vi "TCam_FixpointTemps.vi"(2 "input cluster":T1={"Core"={"Current VI Reference"=refnum, "Close Panel on Exit?"=FALSE}, "Image Out"=refnum, "State"=0, "Points"={"Top Left"={"X"=0.0, "Y"=0.0}, "Top Right"={"X"=0.0, "Y"=0.0}, "Bottom Left"={"X"=0.0, "Y"=0.0}, "Bottom Right"={"X"=0.0, "Y"=0.0}, "x space 2"=0.0, "y space 2"=0.0, "x_space"=0.0, "y_space"=0.0, "Pixels"=[], "Fixpoint"={"X"=0.0, "Y"=0.0}}, "img_array"=[], "Temps"=[], "Temps_Array"=[], "Scan Area"=0.0, "Fixpoint Area"=0.0, "Config"={"Freezing"={"Cutoff"=2.0, "EndIndex"=2}}, "PCR Size"=0, "ImageCount"=0, "ShowGradient"=FALSE, "Save Well data"=FALSE, "Save Blackbody data"=FALSE, "Save Temps For Offset"=FALSE} {"Points"."Bottom Right"."Y" format="%.2f"; "Points"."Bottom Right"."X" format="%.2f"; "Points"."Top Left"."Y" format="%.2f"; "Points"."Top Left"."X" format="%.2f"; "Points"."Top Right"."Y" format="%.2f"; "Points"."Top Right"."X" format="%.2f"; "Points"."Bottom Left"."Y" format="%.2f"; "Points"."Bottom Left"."X" format="%.2f"; "Points"."Fixpoint"."Y" format="%.2f"; "Points"."Fixpoint"."X" format="%.2f"}, 3 "name or relative path":path, 4 "Therm_Temps":dbl[](array[numeric])) -> (0 "WellTemps":dbl[](array[numeric]), 1 "Offsets":dbl[](array[numeric]))   [LabVIEW 2024]
uses:
  DataCluster_TCAL.ctl
  <vilib>/vision/Image Controls.llb/IMAQ Image.ctl
  TCE_Config.ctl
  <vilib>/Utility/file.llb/Write Delimited Spreadsheet (DBL).vi
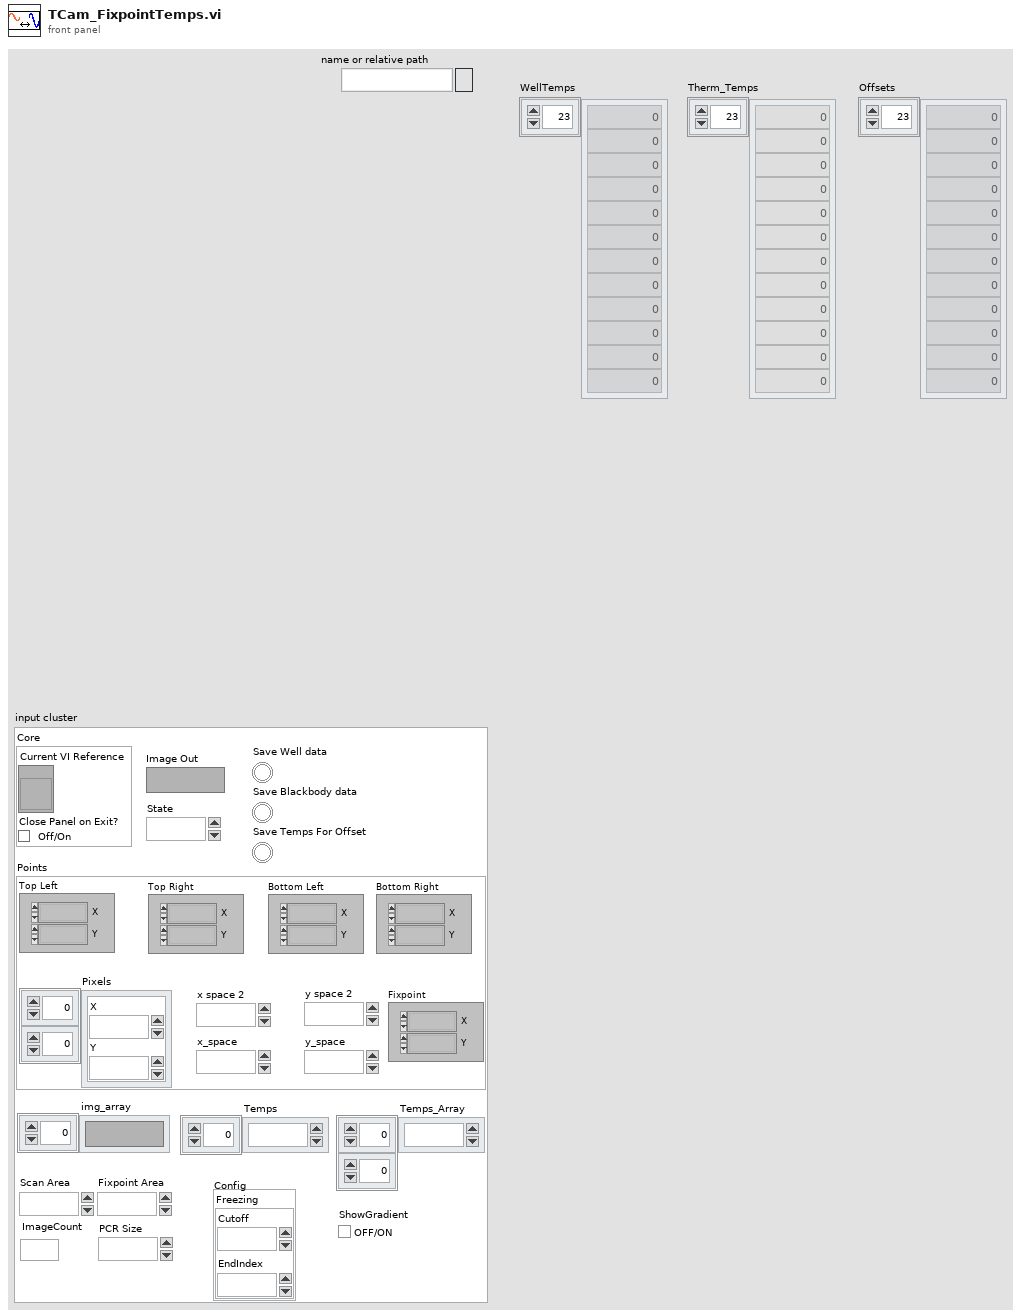
[diagram p1: front panel]
types:
  T1 = typedef "DataCluster_TCAL.ctl" = cluster{"Core":cluster{"Current VI Reference":refnum<vi>, "Close Panel on Exit?":bool}, "Image Out":T2, "State":i32, "Points":cluster{"Top Left":T3, "Top Right":T3, "Bottom Left":T3, "Bottom Right":T3, "x space 2":dbl, "y space 2":sgl, "x_space":sgl, "y_space":sgl, "Pixels":cluster{"X":i32, "Y":i32}[][], "Fixpoint":T3}, "img_array":T2[], "Temps":dbl[], "Temps_Array":dbl[][], "Scan Area":dbl, "Fixpoint Area":dbl, "Config":T4, "PCR Size":u16, "ImageCount":i32, "ShowGradient":bool, "Save Well data":bool, "Save Blackbody data":bool, "Save Temps For Offset":bool}
  T2 = typedef "IMAQ Image.ctl" = refnum<image>
  T3 = typedef "IMAQ Point" = cluster{"X":sgl, "Y":sgl}
  T4 = typedef "TCE_Config.ctl" = cluster{"Freezing":cluster{"Cutoff":dbl, "EndIndex":i32}}
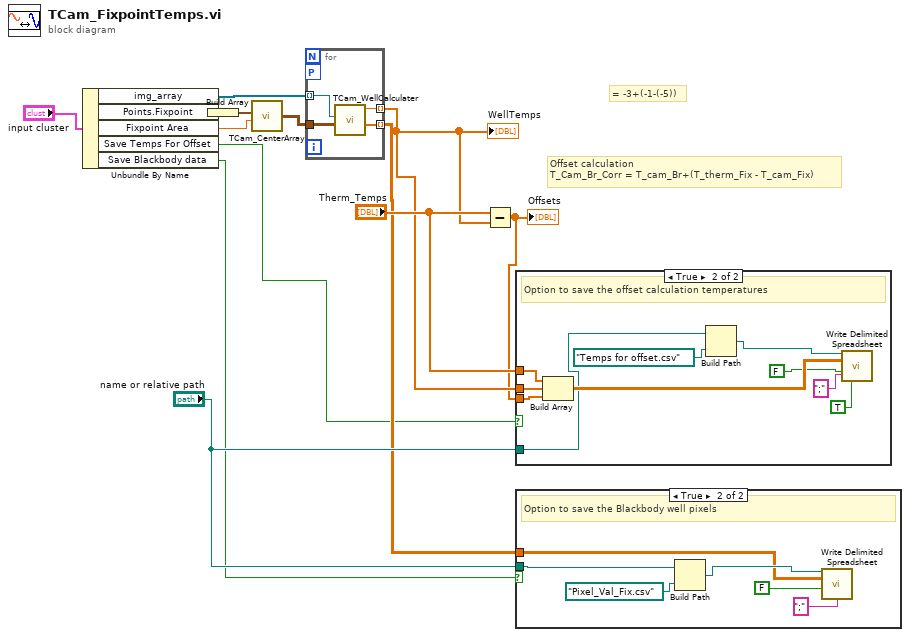
[diagram p0: block diagram]
diagram:
  # "= -3+(-1-(-5))"
  # "Offset calculation\nT_Cam_Br_Corr = T_cam_Br+(T_therm_Fix - T_cam_Fix)"
  n1 = Unbundle By Name("input cluster") -> ("img_array"=w13:T2[], "Points.Fixpoint"=w12:T3, "Fixpoint Area"=w10:dbl, "Save Temps For Offset"=w2:bool, "Save Blackbody data"=w1:bool)
  n2 = Build Array(w12) -> (w11:T3[])
  n3 = call "TCam_CenterArray.vi"("Point Array"=w11, "Size"=w10) -> ("Array"=w9:cluster{"X":i32, "Y":i32}[][])  [unwired: 4 in, 2 out]
  n4 = for {
    tunnel: w13 -> [w16] mode=indexing
    workers-P: _ -> [_]
    tunnel: w9 -> [w17]
    tunnel: [w15] -> w6 mode=indexing
    tunnel: [w14] -> w3 mode=indexing
    n5 = call "TCam_WellCalculater.vi"("Pixels"=w17, "Image in"=w16) -> ("Individual Pixels"=w14:dbl[], "mean"=w15:dbl)  [unwired: 7 in, 1 out]
  }
  "WellTemps" <- w6
  n6 = Subtract(x="Therm_Temps", y=w6) -> (x-y=w5:dbl[])
  "Offsets" <- w5
  n7 = case shown="True" w2 {
    tunnel: w6 -> [_ w24]
    tunnel: "Therm_Temps" -> [_ w25]
    tunnel: w5 -> [_ w21]
    tunnel: "name or relative path" -> [_ w18]
    frame False {
    }
    frame True {
      # "Option to save the offset calculation temperatures"
      n8 = Build Array(w25, w24, w21) -> (w23:dbl[][])
      n9 = Build Path(base path=w18, name or relative path=path "Temps for offset.csv") -> (appended path=w20:path)
      n10 = call-poly <vilib>:"Write Delimited Spreadsheet.vi"("file path (dialog if empty)"=w20, "2D data"=w23, "append to file? (new file:F)"=FALSE ("transpose? (no:F)"), "transpose? (no:F)"=TRUE, "delimiter (\\t)"=";" ("delimiter (\\t)")) -> ()  [unwired: 9 in, 2 out]
    }
  }
  n11 = case shown="True" w1 {
    tunnel: "name or relative path" -> [_ w31]
    tunnel: w3 -> [_ w30]
    frame False {
    }
    frame True {
      # "Option to save the Blackbody well pixels"
      n12 = Build Path(base path=w31, name or relative path=path "Pixel_Val_Fix.csv") -> (appended path=w33:path)
      n13 = call-poly <vilib>:"Write Delimited Spreadsheet.vi"("file path (dialog if empty)"=w33, "2D data"=w30, "append to file? (new file:F)"=FALSE, "delimiter (\\t)"=";" ("delimiter (\\t)")) -> ()  [unwired: 10 in, 2 out]
    }
  }
